vi "锁死与事件响应测试.vi"() -> ()   [LabVIEW 2019, in "test.lvlib"]
uses:
  test.lvlib
panel:
  out "布尔 3":bool
  in  "布尔 2":bool=TRUE
  in  "布尔":bool=TRUE
  in  "簇":cluster{"布尔":bool, "下拉列表":u16, "数组":dbl[]} {"数组" format="%#_13g"}
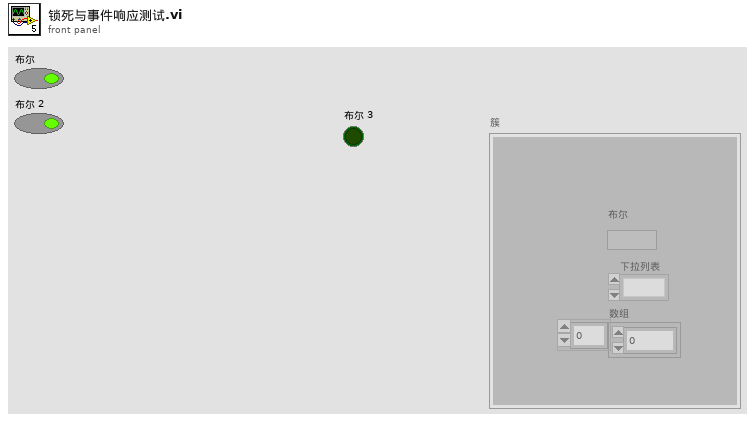
[diagram p1: front panel]
types:
  T1 = enum8{"Enabled", "Disabled", "Disabled and Grayed Out"}
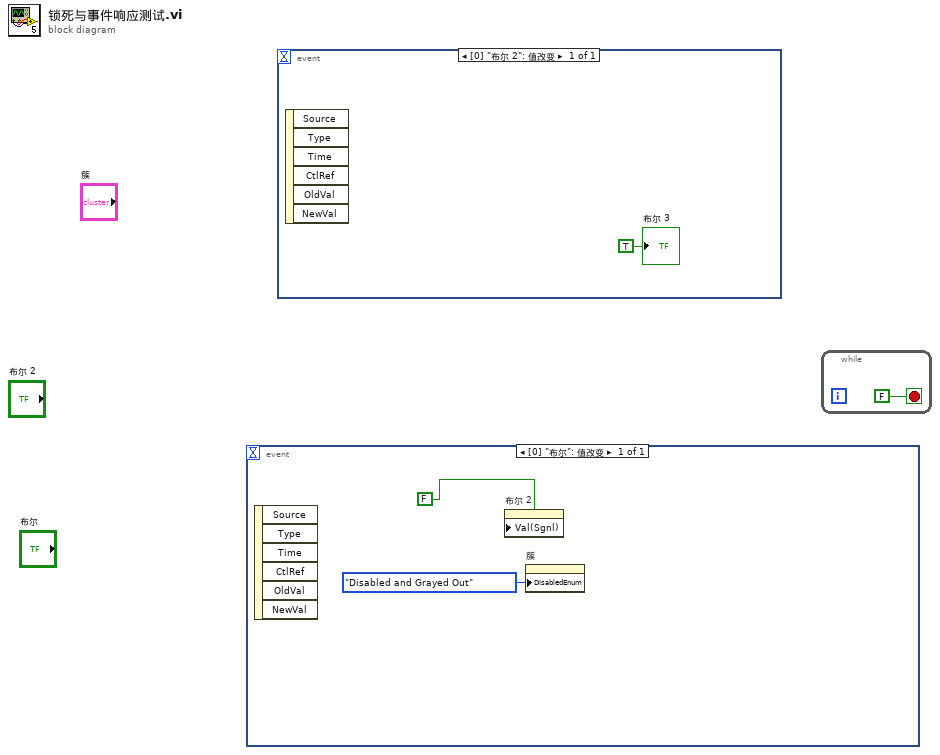
[diagram p0: block diagram]
diagram:
  n1 = event shown="[0] \"布尔\": 值改变" {
    selector: _ -> [_]
    dyn-events: _ -> [_]
    timeout: _ -> [_]
    event "布尔": Value Change {
      n2 = event-data() -> ()  [unwired: 1 in, 6 out]
      n3 = property on="布尔 2" class="Bool (严格)"("Val(Sgnl)"=FALSE ("值(信号)")) -> ()  [unwired: 2 in, 2 out]
      n4 = property on="簇" class="Clust (严格)"("DisabledEnum"=T1."Disabled and Grayed Out" ("禁用")) -> ()  [unwired: 2 in, 2 out]
    }
  }
  n5 = event shown="[0] \"布尔 2\": 值改变" {
    selector: _ -> [_]
    dyn-events: _ -> [_]
    timeout: _ -> [_]
    event "布尔 2": Value Change {
      n6 = event-data() -> ()  [unwired: 1 in, 6 out]
      "布尔 3" <- TRUE ("布尔 3")
    }
  }
  n7 = while {
    stop <- FALSE stop-if-true
  }
